vi "Test Cases - 2D Array in Cluster.vi"() -> ()   [LabVIEW 2017]
uses:
  9f1c8977-aa41-4596-a18a-6dba2ebc59d2.vi
  0333efe5-f0fb-4901-b6dd-db031cec30c6.vi
  API-String-Arugments-Support/_Support/Data To API String Arguments.vi
  API-String-Arugments-Support/_Support/Convert API String Arguments to Data(variant).vi
panel:
  out "String":string
  in  "Cluster":T1={"String"="abc", "BoolArray"=[[TRUE, FALSE, TRUE, FALSE], [FALSE, TRUE, FALSE, TRUE], [TRUE, FALSE, TRUE, FALSE]], "Boolean"=FALSE}
  out "Cluster":T1={"String"="abc", "BoolArray"=[[TRUE, FALSE, TRUE, FALSE], [FALSE, TRUE, FALSE, TRUE], [TRUE, FALSE, TRUE, FALSE]], "Boolean"=FALSE}
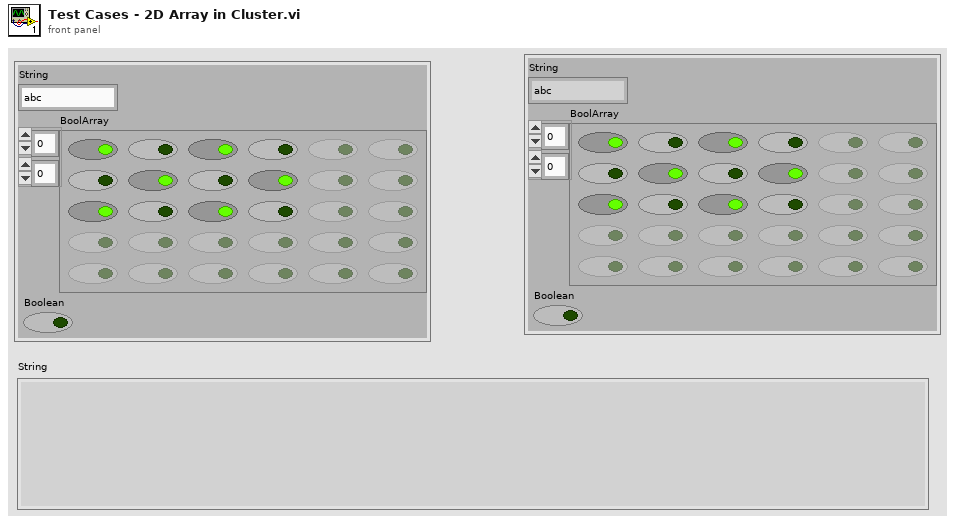
[diagram p1: front panel]
types:
  T1 = cluster{"String":string, "BoolArray":bool[][], "Boolean":bool}
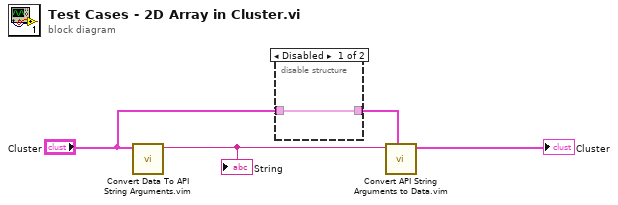
[diagram p0: block diagram]
diagram:
  n1 = call "Convert Data To API String Arguments.vim"("data"="Cluster") -> ("String"=w1:string)  [unwired: 7 in, 1 out]
  "String" <- w1
  n2 = disable-structure "Diagram Disable Structure" shown="Disabled" {
    disable-tunnel: "Cluster" -> [w5 _]
    disable-tunnel: [w5 _] -> w3
    frame Disabled {
    }
    frame Enabled {
    }
  }
  n3 = call "Convert API String Arguments to Data.vim"("Type"=w3, "String"=w1) -> ("Data"=→"Cluster":T1)  [unwired: 6 in, 1 out]
